vi "Get Socket My Index.vi"(8 "error in (no error)":errorcluster, 11 "Teststand in":refnum<class "Teststand.lvclass">) -> (0 "error out":errorcluster, 2 "Socket":i16, 3 "Teststand out":refnum<class "Teststand.lvclass">)   [LabVIEW 2023, in "HardwareAbstractionLayer_LVOOP.lvlib" / "Teststand.lvclass"]
uses:
  Teststand.lvclass
  Teststand.lvclass/Teststand.ctl
  <vilib>/addons/TestStand/_TSUtility.llb/TestStand - Get Property Value (Number {Signed 16-bit Integer}).vi
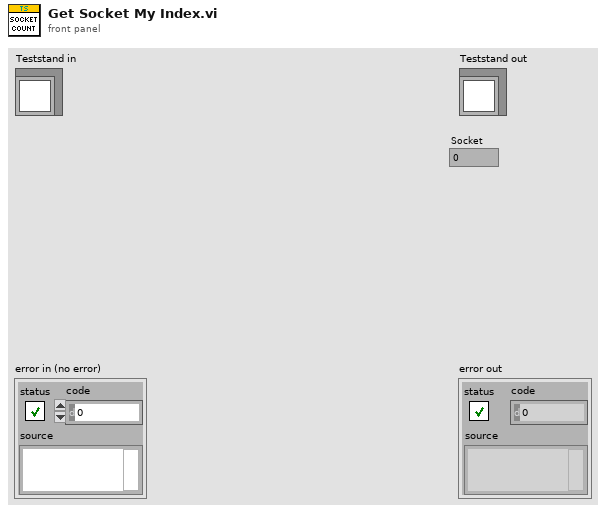
[diagram p1: front panel]
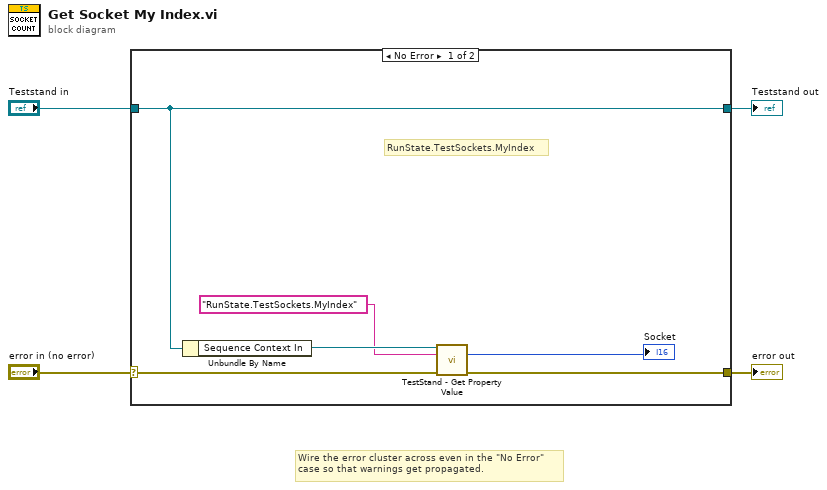
[diagram p0: block diagram]
diagram:
  # "Wire the error cluster across even in the \"No Error\"\ncase so that warnings get propagated."
  n1 = case shown="No Error" "error in (no error)" {
    selector: "error in (no error)" -> [w8 w12]
    tunnel: [w7 w12] -> w3
    tunnel: [w10 w11] -> w1
    tunnel: "Teststand in" -> [w10 w11]
    frame No Error {
      # "RunState.TestSockets.MyIndex"
      n2 = Unbundle By Name(w10) -> ("Sequence Context In"=w9:refnum<k7>)
      n3 = call-poly <vilib>:"TestStand - Get Property Value.vi"("Sequence Context In"=w9, "Lookup String"="RunState.TestSockets.MyIndex", "error in (no error)"=w8) -> ("Value"=→"Socket":i16, "error out"=w7:errorcluster)  [unwired: 10 in, 1 out]
    }
    frame Error {
    }
  }
  "error out" <- w3
  "Teststand out" <- w1
